vi "RobotDriveMecanumDrive_Cartesian.vi"(5 "Motor Modifiers":T1, 6 "Rotation":dbl, 7 "Gyro Angle":dbl, 8 "error in (no error)":errorcluster, 9 "Y":dbl, 10 "X":dbl, 11 "RobotDriveDevRef":T2={"DevStatus"={"status"=FALSE, "code"=0, "source"=""}, "Motors[]"=[], "Square Inputs"=FALSE, "Max Output"=1.0}) -> (0 "error out":errorcluster, 2 "Motor Values":dbl[](array[numeric]), 3 "RobotDriveDevRef":T2={"DevStatus"={"status"=FALSE, "code"=0, "source"=""}, "Motors[]"=[], "Square Inputs"=FALSE, "Max Output"=1.0})   [LabVIEW 2014]
doc: "Configures the motors for holonomic driving. Holonomic driving allows you to move the robot in any direction without first rotating or maneuvering the robot.\n\nThis VI requires the robot to have either four omni-directional wheels and four motors mounted at 45 degree angles in the four corners of a square frame or to have four mecanum wheels driven by four motors.\n\nThe control input is intended to be connected directly to the X, Y, and Z axes of a joystick. The Y axis is inverted for you.\n\nThis software is licensed. Open the labview\\readme\\WPI Robotics Library Open Source License.txt file for more information."
uses:
  <vilib>/Rock Robotics/WPI/RobotDrive/WPI_RobotDriveDevRef.ctl
  <vilib>/Rock Robotics/WPI/MotorControl/WPI_MotorControlDeviceRef.ctl
  <vilib>/Rock Robotics/WPI/MotorControl/WPI_MotorControlType.ctl
  <vilib>/Rock Robotics/SystemInterfaces/Typedef/FPGA_TypedefDigitalModule.ctl
  <vilib>/Rock Robotics/SystemInterfaces/DIO/FPGA_DIOPWMChannel.ctl
  <vilib>/Rock Robotics/WPI/PWM/WPI_PWMDeadband.ctl
  <vilib>/Rock Robotics/WPI/CAN/Jaguar/SubVIs/WPI_CANJaguar_ControlMode.ctl
  <vilib>/Rock Robotics/WPI/CAN/TalonSRX/WPI_CANTalonSRX_APIControlMode.ctl
  <vilib>/Rock Robotics/WPI/PWM/WPI_PWMTransform_ConPane.ctl
  <vilib>/Rock Robotics/SystemInterfaces/NetworkCommunication/NetComm_UsageReport_ResourceType.ctl
  <vilib>/Rock Robotics/WPI/RobotDrive/WPI_RobotDriveMotorSelectorEnum.ctl
  <vilib>/Rock Robotics/WPI/RobotDrive/WPI_RobotDriveSafetyCheck.vi
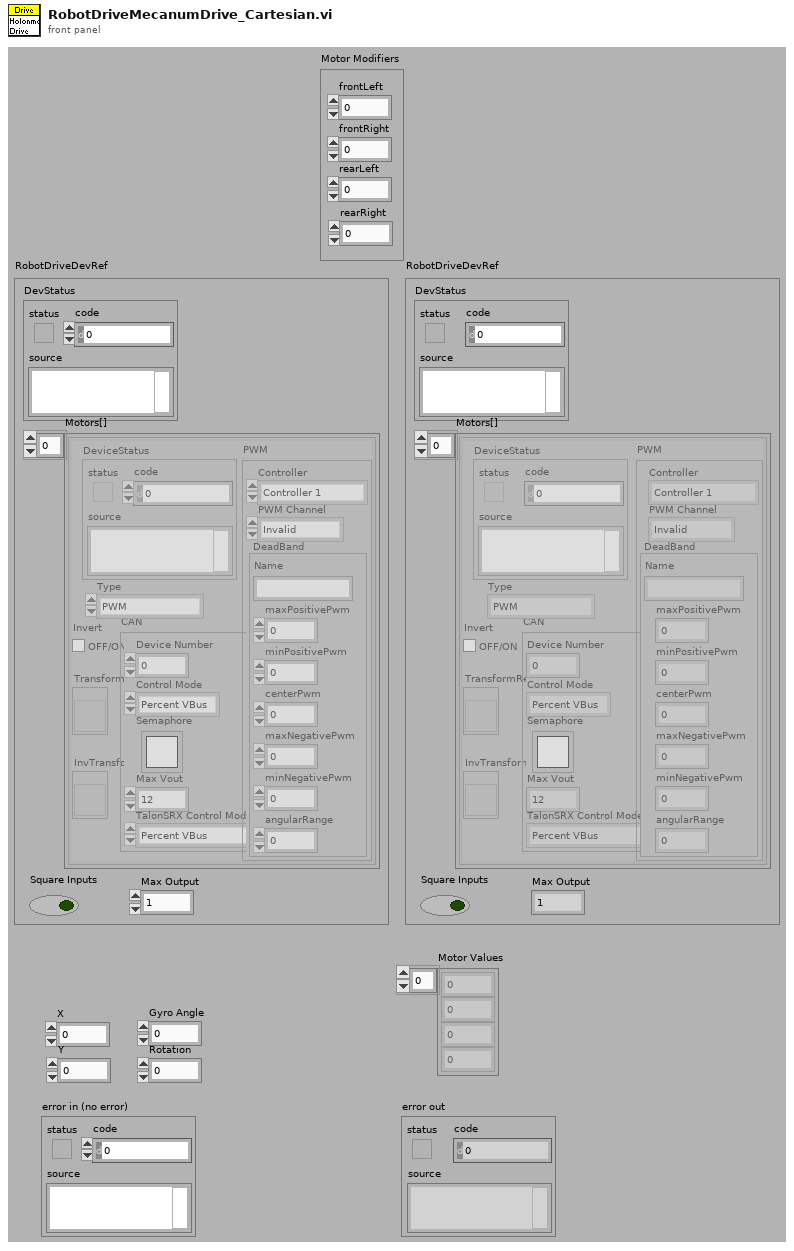
[diagram p1: front panel]
types:
  T1 = cluster{"frontLeft":dbl, "frontRight":dbl, "rearLeft":dbl, "rearRight":dbl}
  T2 = typedef "WPI_RobotDriveDevRef.ctl" = cluster{"DevStatus":errorcluster, "Motors[]":T3[], "Square Inputs":bool, "Max Output":dbl}
  T3 = typedef "WPI_MotorControlDeviceRef.ctl" = cluster{"DeviceStatus":errorcluster, "Type":T4, "PWM":cluster{"Controller":T5, "PWM Channel":T6, "DeadBand":T7}, "CAN":cluster{"Device Number":u8, "Control Mode":T8, "Semaphore":T9, "Max Vout":dbl, "TalonSRX Control Mode":T10}, "Invert":bool, "TransformRef":T11, "InvTransformRef":T11}
  T4 = typedef "WPI_MotorControlType.ctl" = enum16{"PWM", "CAN", "CANTalonSRX"}
  T5 = typedef "FPGA_TypedefDigitalModule.ctl" = enum16{"Controller 1"}
  T6 = typedef "FPGA_DIOPWMChannel.ctl" = enum8{"PWM 0", "PWM 1", "PWM 2", "PWM 3", "PWM 4", "PWM 5", "PWM 6", "PWM 7", "PWM 8", "PWM 9", "PWM MXP 0", "PWM MXP 1", "PWM MXP 2", "PWM MXP 3", "PWM MXP 4", "PWM MXP 5", "PWM MXP 6", "PWM MXP 7", "PWM MXP 8", "PWM MXP 9", "Invalid"}
  T7 = typedef "WPI_PWMDeadband.ctl" = cluster{"Name":string, "maxPositivePwm":i32, "minPositivePwm":i32, "centerPwm":i32, "maxNegativePwm":i32, "minNegativePwm":i32, "angularRange":u16}
  T8 = typedef "WPI_CANJaguar_ControlMode.ctl" = enum8{"Percent VBus", "Current", "Speed", "Position", "Voltage"}
  T9 = typedef "Semaphore RefNum" = refnum<k1>
  T10 = typedef "WPI_CANTalonSRX_APIControlMode.ctl" = enum8{"Percent VBus", "Speed", "Position", "Slave", "Unchanged / Invalid"}
  T11 = typedef "WPI_PWMTransform_ConPane.ctl" = refnum<vi>
  T12 = typedef "NetComm_UsageReport_ResourceType.ctl" = enum8{"Controller", "Module", "Language", "CANPlugin", "Accelerometer", "ADXL345", "AnalogChannel", "AnalogTrigger", "AnalogTriggerOutput", "CANJaguar", "Compressor", "Counter", "Dashboard", "DigitalInput", "DigitalOutput", "DriverStationCIO", "DriverStationEIO", "DriverStationLCD", "Encoder", "GearTooth", "Gyro", "I2C", "Framework", "Jaguar", "Joystick", "Kinect", "KinectStick", "PIDController", "Preferences", "PWM", "Relay", "RobotDrive", "SerialPort", "Servo", "Solenoid", "SPI", "Task", "Ultrasonic", "Victor", "Button", "Command", "AxisCamera", "PCVideoServer", "SmartDashboard", "Talon", "HiTechnicColorSensor", "HiTechnicAccel", "HiTechnicCompass", "SRF08", "AnalogOutput", "Victor SP", "Talon SRX", "CAN Talon SRX"}
  T13 = typedef "WPI_RobotDriveMotorSelectorEnum.ctl" = enum16{"Rear Left Motor", "Rear Right Motor", "Front Left Motor", "Front Right Motor"}
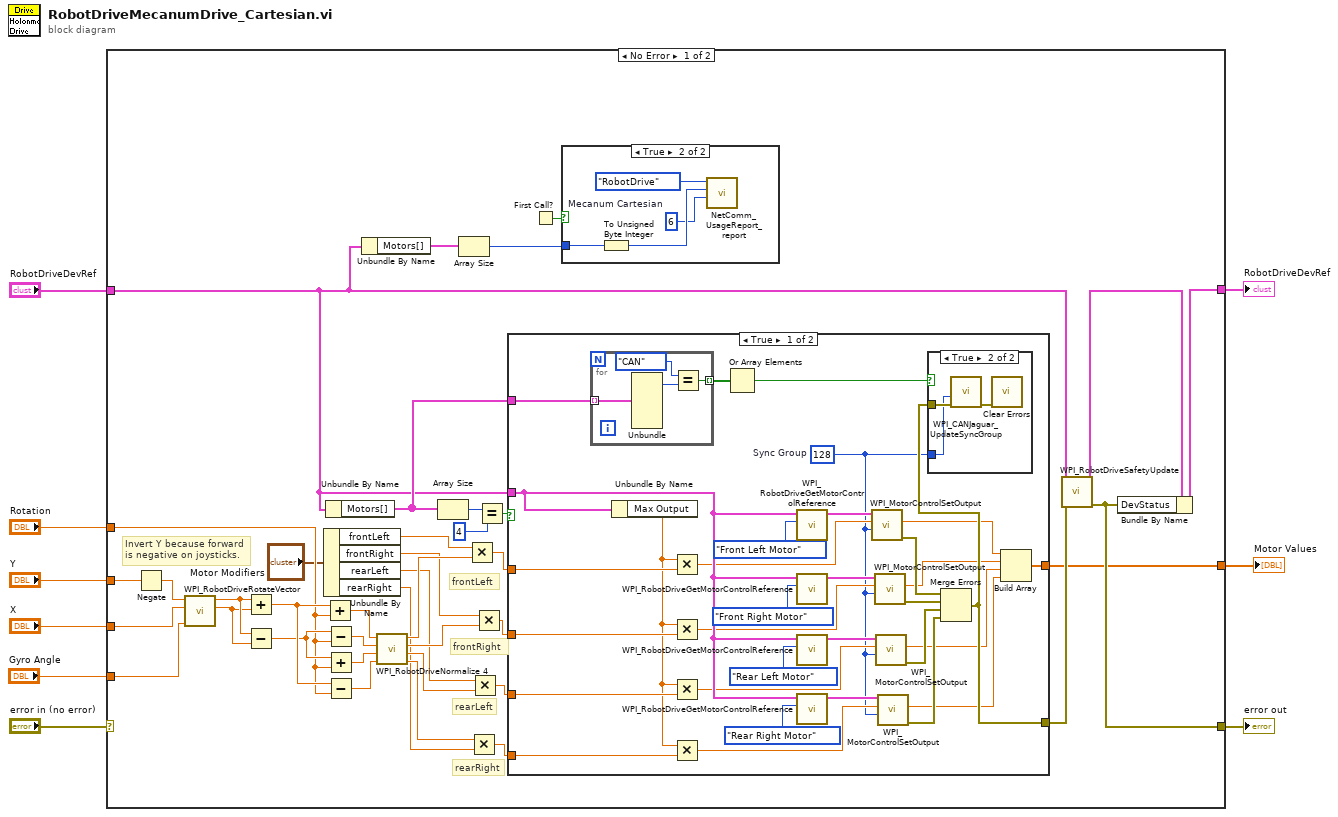
[diagram p0: block diagram]
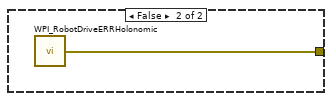
[diagram p4: hidden frame]
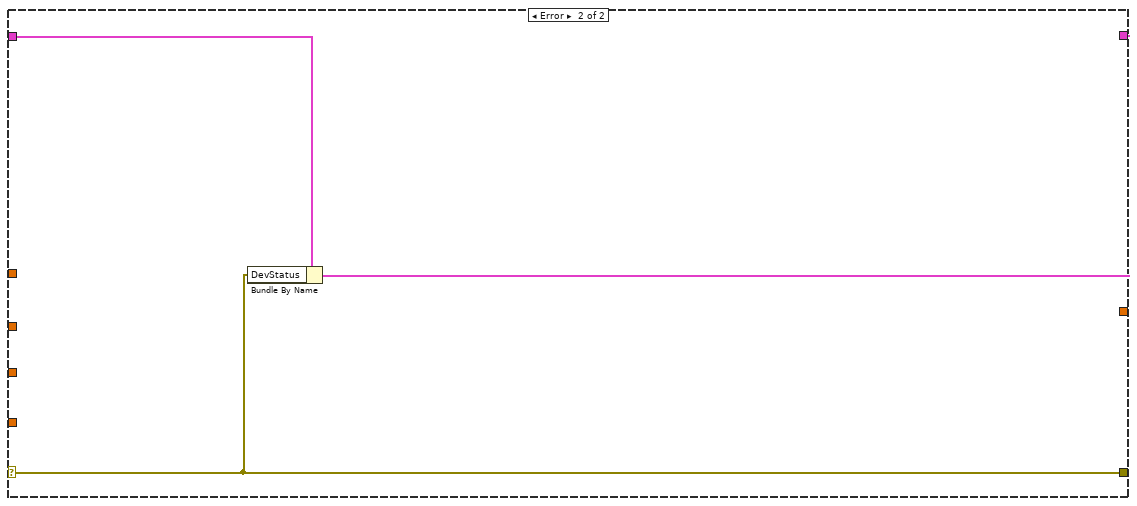
[diagram p5: hidden frame]
diagram:
  n1 = case shown="No Error" "error in (no error)" {
    selector: "error in (no error)" -> [_ w93]
    tunnel: "Y" -> [w30 _]
    tunnel: "X" -> [w35 _]
    tunnel: "RobotDriveDevRef" -> [w20 w95]
    tunnel: [w45 w94] -> w5
    tunnel: [w25 w93] -> w4
    tunnel: "Rotation" -> [w36 _]
    tunnel: "Gyro Angle" -> [w29 _]
    tunnel: [w19 _] -> w1
    frame No Error {
      # "Invert Y because forward is negative on joysticks."
      # "rearLeft"
      # "frontRight"
      # "rearRight"
      # "frontLeft"
      n2 = Negate(x=w30) -> (-x=w28:dbl)
      n3 = call <vilib>:"WPI_RobotDriveRotateVector.vi"("Angle"=w29, "X"=w35, "Y"=w28) -> ("X'"=w43:dbl, "Y'"=w44:dbl)  [unwired: 7 out]
      n4 = Add(x=w44, y=w43) -> (x+y=w41:dbl)
      n5 = Subtract(x=w44, y=w43) -> (x-y=w39:dbl)
      n6 = Unbundle By Name("Motor Modifiers") -> ("frontLeft"=w13:dbl, "frontRight"=w12:dbl, "rearLeft"=w11:dbl, "rearRight"=w10:dbl)
      n7 = Add(x=w41, y=w36) -> (x+y=w37:dbl)
      n8 = Unbundle By Name(w20) -> ("Motors[]"=w24:T3[])
      n9 = Subtract(x=w39, y=w36) -> (x-y=w38:dbl)
      n10 = Add(x=w39, y=w36) -> (x+y=w40:dbl)
      n11 = Subtract(x=w41, y=w36) -> (x-y=w42:dbl)
      n12 = Unbundle By Name(w20) -> ("Motors[]"=w22:T3[])
      n13 = call <vilib>:"WPI_RobotDriveNormalize 4.vi"("D"=w42, "C"=w40, "B"=w38, "A"=w37) -> ("D'"=w32:dbl, "C'"=w31:dbl, "B'"=w33:dbl, "A'"=w34:dbl)
      n14 = Array Size(array=w24) -> (size(s)=w48:i32)
      n15 = Array Size(array=w22) -> (size(s)=w21:i32)
      n16 = Multiply(x=w13, y=w34) -> (x*y=w18:dbl)
      n17 = Multiply(x=w32, y=w10) -> (x*y=w15:dbl)
      n18 = Multiply(x=w11, y=w31) -> (x*y=w16:dbl)
      n19 = Multiply(x=w12, y=w33) -> (x*y=w17:dbl)
      n20 = Equal?(x=w48, y=4) -> (x = y?=w46:bool)
      n21 = case shown="True" w46 {
        tunnel: w18 -> [w84 _]
        tunnel: w17 -> [w83 _]
        tunnel: w20 -> [w72 _]
        tunnel: [w59 w92] -> w27
        tunnel: w16 -> [w78 _]
        tunnel: w15 -> [w77 _]
        tunnel: w24 -> [w60 _]
        tunnel: [w56 _] -> w19
        frame True {
          w58 = u8 128  # Sync Group
          n22 = for {
            tunnel: w60 -> [w88] mode=indexing
            tunnel: [w85] -> w61 mode=indexing
            n23 = Unbundle(w88) -> ("Type"=w87:T4)  [unwired: 6 out]
            n24 = Equal?(x=enum16{"PWM", "CAN"}."CAN" ("Type"), y=w87) -> (x = y?=w85:bool)
          }
          n25 = Unbundle By Name(w72) -> ("Max Output"=w67:dbl)
          n26 = Multiply(x=w67, y=w84) -> (x*y=w71:dbl)
          n27 = Multiply(x=w67, y=w83) -> (x*y=w70:dbl)
          n28 = Multiply(x=w67, y=w78) -> (x*y=w69:dbl)
          n29 = Multiply(x=w67, y=w77) -> (x*y=w68:dbl)
          n30 = Or Array Elements(Boolean array=w61) -> (logical OR=w62:bool)
          n31 = call <vilib>:"WPI_RobotDriveGetMotorControlReference.vi"("MotorIndex"=WPI_RobotDriveMotorSelectorEnum."Front Left Motor", "RobotDriveDevRef"=w72) -> ("MotorControlDeviceRef"=w82:T3)  [unwired: 9 out]
          n32 = call <vilib>:"WPI_RobotDriveGetMotorControlReference.vi"("MotorIndex"=WPI_RobotDriveMotorSelectorEnum."Front Right Motor", "RobotDriveDevRef"=w72) -> ("MotorControlDeviceRef"=w80:T3)  [unwired: 9 out]
          n33 = call <vilib>:"WPI_RobotDriveGetMotorControlReference.vi"("MotorIndex"=WPI_RobotDriveMotorSelectorEnum."Rear Left Motor", "RobotDriveDevRef"=w72) -> ("MotorControlDeviceRef"=w81:T3)  [unwired: 9 out]
          n34 = call <vilib>:"WPI_RobotDriveGetMotorControlReference.vi"("MotorIndex"=WPI_RobotDriveMotorSelectorEnum."Rear Right Motor", "RobotDriveDevRef"=w72) -> ("MotorControlDeviceRef"=w79:T3)  [unwired: 9 out]
          n35 = call <vilib>:"WPI_MotorControlSetOutput.vi"("Sync Group / Parameter Slot"=w58, "Output"=w71, "MotorControlDevRef"=w82) -> ("error out"=w63:errorcluster, "Motor Output"=w57:dbl)  [unwired: 2 in, 5 out]
          n36 = call <vilib>:"WPI_MotorControlSetOutput.vi"("Sync Group / Parameter Slot"=w58, "Output"=w70, "MotorControlDevRef"=w80) -> ("error out"=w64:errorcluster, "Motor Output"=w55:dbl)  [unwired: 2 in, 5 out]
          n37 = call <vilib>:"WPI_MotorControlSetOutput.vi"("Sync Group / Parameter Slot"=w58, "Output"=w69, "MotorControlDevRef"=w81) -> ("error out"=w65:errorcluster, "Motor Output"=w54:dbl)  [unwired: 2 in, 5 out]
          n38 = call <vilib>:"WPI_MotorControlSetOutput.vi"("Sync Group / Parameter Slot"=w58, "Output"=w68, "MotorControlDevRef"=w79) -> ("error out"=w66:errorcluster, "Motor Output"=w53:dbl)  [unwired: 2 in, 5 out]
          n39 = Merge Errors(w63, w64, w65, w66) -> (w59:errorcluster)
          n40 = case shown="True" w62 {
            tunnel: w59 -> [_ w90]
            tunnel: w58 -> [_ w89]
            frame False {
            }
            frame True {
              n41 = call <vilib>:"WPI_CANJaguar_UpdateSyncGroup.vi"("error in (no error)"=w90, "Sync Group"=w89) -> ("error out"=w91:errorcluster)  [unwired: 9 out]
              n42 = call <vilib>:"Clear Errors.vi"("error in (no error)"=w91) -> ()  [unwired: 1 in, 6 out]
            }
          }
          n43 = Build Array(w57, w55, w54, w53) -> (w56:dbl[])
        }
        frame False {
          n44 = call <vilib>:"WPI_RobotDriveERRHolonomic.vi"() -> ("error out"=w92:errorcluster)
        }
      }
      n45 = First Call?() -> (First Call?: T/F=w23:bool)
      n46 = case shown="True" w23 {
        tunnel: w21 -> [_ w51]
        frame False {
        }
        frame True {
          w49 = u8 6  # Mecanum Cartesian
          n47 = To Unsigned Byte Integer(number=w51) -> (unsigned 8bit integer=w50:u8)
          n48 = call <vilib>:"NetComm_UsageReport_report.vi"("Context"=w49, "Instance Number"=w50, "Resource Type"=NetComm_UsageReport_ResourceType."RobotDrive") -> ()  [unwired: 9 in]
        }
      }
      n49 = call <vilib>:"WPI_RobotDriveSafetyUpdate.vi"("error in (no error)"=w27, "RobotDriveDevRef"=w20) -> ("error out"=w25:errorcluster, "RobotDriveDevRef"=w26:T2)  [unwired: 8 out]
      n50 = Bundle By Name(cluster=w26, "DevStatus"=w25) -> (w45:T2)
    }
    frame Error {
      n51 = Bundle By Name(cluster=w95, "DevStatus"=w93) -> (w94:T2)
    }
  }
  "error out" <- w4
  "RobotDriveDevRef" <- w5
  "Motor Values" <- w1
